vi "U8-Array-to-U64-Array.vi"(11 "Frame U8[] in":u8[](array[numeric]) format="%.0x") -> (3 "Frame U64[] out":u64[](array[numeric]) format="%.0x")   [LabVIEW 2017]
panel:
  out "Grid View\n(for Debug Purposes)":u8[][](array[numeric]) format="%.0x"
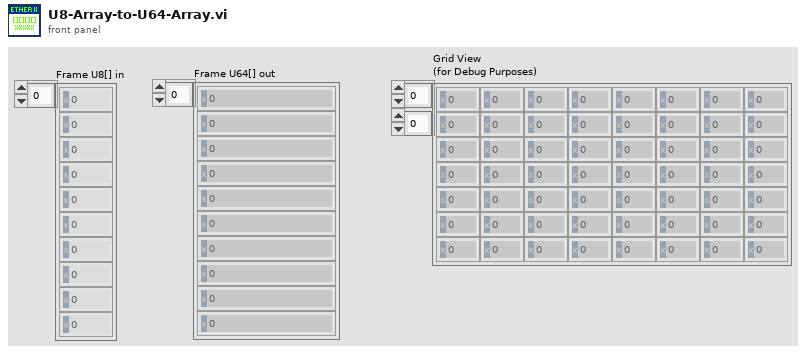
[diagram p1: front panel]
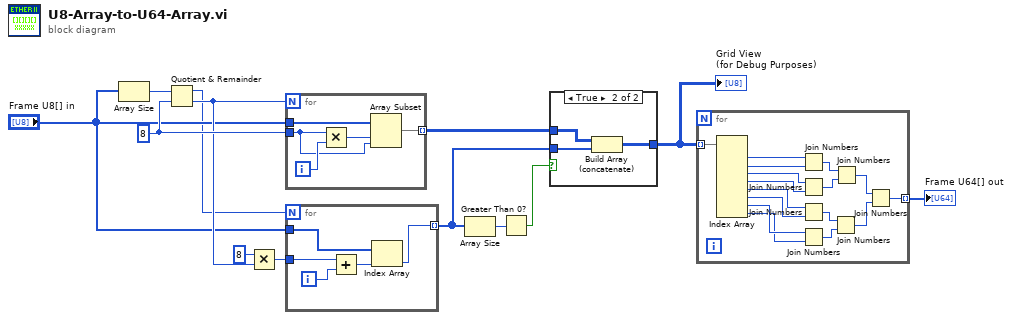
[diagram p0: block diagram]
diagram:
  w12 = 8 ("y")
  n1 = Array Size(array="Frame U8[] in") -> (size(s)=w13:i32)
  n2 = Quotient & Remainder(x=w13, y=w12) -> (x-y*floor(x/y)=w5:i32, floor(x/y)=w7:i32)
  n3 = Multiply(x=8, y=w7) -> (x*y=w9:i32)
  n4 = for {
    N: w7 -> [_]
    tunnel: w12 -> [w16]
    tunnel: [w14] -> w11 mode=indexing
    tunnel: "Frame U8[] in" -> [w15]
    i -> [w17]
    n5 = Multiply(x=w16, y=w17) -> (x*y=w18:i32)
    n6 = Array Subset(array=w15, index=w18, length=w16) -> (w14:u8[])
  }
  n7 = for {
    N: w5 -> [_]
    tunnel: w9 -> [w21]
    tunnel: "Frame U8[] in" -> [w20]
    tunnel: [w19] -> w3 mode=indexing
    i -> [w22]
    n8 = Add(x=w21, y=w22) -> (x+y=w23:i32)
    n9 = Index Array(array=w20, index=w23) -> (element=w19:u8)
  }
  n10 = Array Size(array=w3) -> (size(s)=w2:i32)
  n11 = Greater Than 0?(x=w2) -> (x > 0?=w1:bool)
  n12 = case shown="True" w1 {
    tunnel: w11 -> [w24 w27]
    tunnel: [w24 w26] -> w4
    tunnel: w3 -> [_ w25]
    frame False {
    }
    frame True {
      n13 = Build Array (concatenate)(w27, w25) -> (w26:u8[][])
    }
  }
  "Grid View\n(for Debug Purposes)" <- w4
  n14 = for {
    tunnel: w4 -> [w43] mode=indexing
    tunnel: [w28] -> w10 mode=indexing
    n15 = Index Array(array=w43) -> (element #1=w42:u8, element #2=w41:u8, element #3=w40:u8, element #4=w39:u8, element #5=w38:u8, element #6=w37:u8, element #7=w36:u8, element #8=w35:u8)  [unwired: 8 in]
    n16 = Join Numbers(hi=w42, lo=w41) -> ((hi.lo)=w34:u16)
    n17 = Join Numbers(hi=w40, lo=w39) -> ((hi.lo)=w33:u16)
    n18 = Join Numbers(hi=w38, lo=w37) -> ((hi.lo)=w32:u16)
    n19 = Join Numbers(hi=w36, lo=w35) -> ((hi.lo)=w31:u16)
    n20 = Join Numbers(hi=w32, lo=w31) -> ((hi.lo)=w30:u32)
    n21 = Join Numbers(hi=w34, lo=w33) -> ((hi.lo)=w29:u32)
    n22 = Join Numbers(hi=w29, lo=w30) -> ((hi.lo)=w28:u64)
  }
  "Frame U64[] out" <- w10
